vi "Initial MovCor bundler-DBL.vi"(8 "error in (no error)":errorcluster, 9 "Ini file interface":T2, 10 "Section name":string, 11 "Setup.ini ref":T1) -> (0 "error out":errorcluster, 3 "Setup.ini ref":T1)   [LabVIEW 2017]
uses:
  Typedefs/Ini file interface (DBL).ctl
  <vilib>/Utility/config.llb/Config Data RefNum.ctl
  <vilib>/Utility/config.llb/NI_LVConfig.lvlib
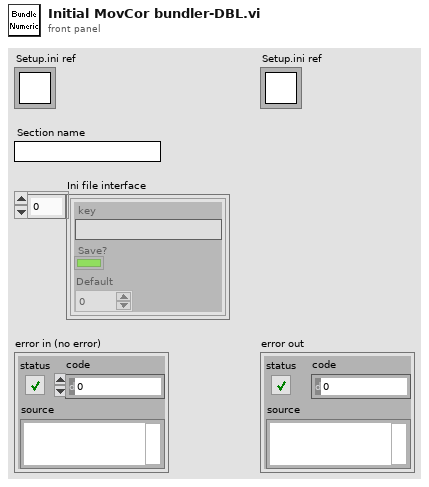
[diagram p1: front panel]
types:
  T1 = typedef "NI_LVConfig.lvlib/Config Data RefNum.ctl" = refnum<k1>
  T2 = typedef "Ini file interface (DBL).ctl" = cluster{"key":string, "Save?":bool, "Default":dbl}[]
  T3 = typedef "Ref DAQ Param.ctl" = cluster{"Full Frame Size":u16, "Ref Field of View":sgl, "Ref Zoom":i8, "Ref_dwellTime":sgl, "Ref X-pixels-per-line(Npxr)":i16, "Ref Y-lines-per-image(Npyr)":i16, "Ref Z-lines-per-image":i16, "Ref Scan Cycles":i32, "Ref threshold":u16, "Ref average":u16, "Sliding Average":bool, "proportioanl_scale":fxp<+,16,2>, "Integral_scale":fxp<+/-,16,12>, "proportioanl_scaleZ":fxp<+,16,2>, "Integral_scaleZ":fxp<+/-,16,12>, "Diff_threshold":fxp<+,16,2>, "Diff_threshold _z":fxp<+,16,2>, "scale":fxp<+,16,2>, "Control algorithm":T4, "New line trigger enabled":bool, "Slide Averaging":bool, "Ref count reset enabled":bool}
  T4 = typedef "Control algorithm.ctl" = enum16{"PID", "Kalman"}
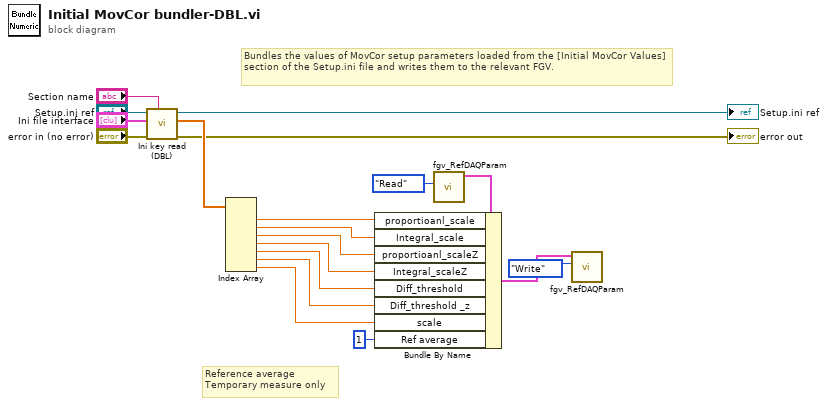
[diagram p0: block diagram]
diagram:
  # "Reference average\nTemporary measure only"
  # "Bundles the values of MovCor setup parameters loaded from the [Initial MovCor Values] section of the Setup.ini file and writes them to the relevant FGV."
  n1 = call "Ini key read (DBL).vi"("Section name"="Section name", "error in (no error)"="error in (no error)", "Parameter names & setup"="Ini file interface", "Ini file refnum in"="Setup.ini ref") -> ("error out"=→"error out":errorcluster, "Value read/used"=w13:dbl[], "Ini file refnum out"=→"Setup.ini ref":T1)  [unwired: 5 in]
  n2 = Index Array(array=w13) -> (element #1=w8:dbl, element #2=w7:dbl, element #3=w6:dbl, element #4=w5:dbl, element #5=w4:dbl, element #6=w3:dbl, element #7=w2:dbl)  [unwired: 7 in]
  n3 = call "fgv_RefDAQParam.vi"("Function"=enum16{"Initialize", "Write", "Read"}."Read") -> ("RefDAQParam"=w19:T3)  [unwired: 9 in, 1 out]
  n4 = Bundle By Name(cluster=w19, "proportioanl_scale"=w8, "Integral_scale"=w7, "proportioanl_scaleZ"=w6, "Integral_scaleZ"=w5, "Diff_threshold"=w4, "Diff_threshold _z"=w3, "scale"=w2, "Ref average"=u16 1) -> (w17:T3)
  n5 = call "fgv_RefDAQParam.vi"("Function"=enum16{"Initialize", "Write", "Read"}."Write" ("Status"), "RefDAQParam in"=w17) -> ()  [unwired: 8 in, 2 out]
